vi "ErrorCodes (SubVI).vi"(8 "error in (no error)":errorcluster, 11 "Input":string) -> (0 "error out":errorcluster)   [LabVIEW 2018]
uses:
  <vilib>/regexp/Match Regular Expression.xnode
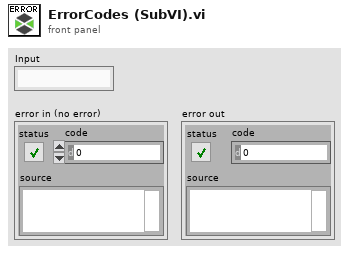
[diagram p1: front panel]
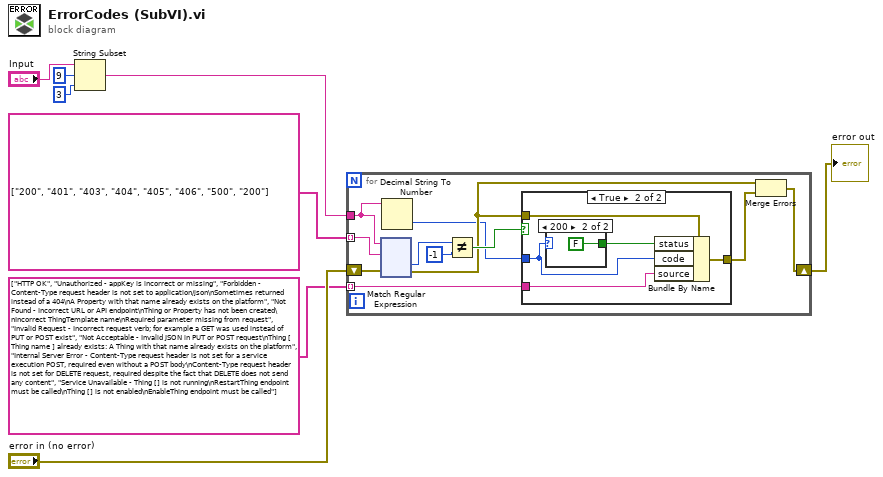
[diagram p0: block diagram]
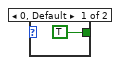
[diagram p3: hidden frame]
diagram:
  n1 = String Subset(string="Input", offset (0)=9, length (rest)=3 ("length (rest)")) -> (substring=w3:string)
  n2 = for {
    tunnel: w3 -> [w12]
    tunnel: string[] ["200", "401", "403", "404", "405", "406", "500", "200"] -> [w17] mode=indexing
    tunnel: string[] ["HTTP OK", "Unauthorized - appKey is incorrect or missing", "Forbidden - Content-Type request header is not set to application/json\nSometimes returned instead of a 404\nA Property with that name already exists on the platform", "Not Found - Incorrect URL or API endpoint\nThing or Property has not been created\nIncorrect ThingTemplate name\nRequired parameter missing from request", "Invalid Request - Incorrect request verb; for example a GET was used instead of PUT or POST exist", "Not Acceptable - Invalid JSON in PUT or POST request\nThing [ Thing name ] already exists: A Thing with that name already exists on the platform", "Internal Server Error - Content-Type request header is not set for a service execution POST, required even without a POST body\nContent-Type request header is not set for DELETE request, required despite the fact that DELETE does not send any content", "Service Unavailable - Thing [] is not running\nRestartThing endpoint must be called\nThing [] is not enabled\nEnableThing endpoint must be called"] -> [w10] mode=indexing
    shift-right: [w9] -> w1
    shift-left: "error in (no error)" -> [w16]
    n3 = xnode "Match Regular Expression"("input string"=w12, "regular expression"=w17, "error in"=w16) -> ("offset past match"=w19:i32, "error out"=w13:errorcluster)  [unwired: 3 in, 3 out]
    n4 = Decimal String To Number(string=w12) -> (number=w11:i32)  [unwired: 2 in, 1 out]
    n5 = Not Equal?(x=w19, y=-1) -> (x != y?=w14:bool)
    n6 = case shown="True" w14 {
      tunnel: w13 -> [w20 w25]
      tunnel: [w20 w24] -> w15
      tunnel: w10 -> [_ w23]
      tunnel: w11 -> [_ w22]
      frame False {
      }
      frame True {
        n7 = case shown="200" w22 {
          tunnel: [TRUE ("status") FALSE ("status")] -> w21
          frame 0, Default {
          }
          frame 200 {
          }
        }
        n8 = Bundle By Name(cluster=w25, "status"=w21, "code"=w22, "source"=w23) -> (w24:errorcluster)
      }
    }
    n9 = Merge Errors(w13, w15) -> (w9:errorcluster)
  }
  "error out" <- w1
